vi "CPP-Multiplot.vi"(0 "PlotArray":cluster{dbl[], dbl[]}[](array[cluster]), 1 "Job Directory":path) -> (2 "Saved Automatically?":bool, 3 "gnuplotScript":string, 4 "Plot data file":path)   [LabVIEW 2014]
uses:
  gnuplotScriptComponents/plotstyle.ctl
  gnuplotScriptComponents/graphPeripherals.ctl
  gnuplotScriptComponents/minAndMax.ctl
  gnuplotScriptComponents/AutoManualNumber.ctl
  gnuplotScriptComponents/ticsAndGrids.ctl
  gnuplotScriptComponents/tics.ctl
  gnuplotScriptComponents/grids.ctl
  gnuplotScriptComponents/legendProperties.ctl
  gnuplotScriptComponents/legendAppearance.ctl
  gnuplotScriptComponents/alignment.ctl
  gnuplotScriptComponents/at.ctl
  gnuplotScriptComponents/margins.ctl
  gnuplotScriptComponents/source.ctl
  gnuplotScriptComponents/Master_Legend.ctl
  gnuplotScriptComponents/MasterPeripherals.ctl
  gnuplotScriptComponents/axisName.ctl
  Results_plotter_Global.vi
panel:
  out "Multi_Plot":bool
  in  "OpenLogfile?":bool
  in  "Show Script Editor?":bool
  in  "Tab Control":T1(tab)=enum."Appearance"
  in  "Each Graph contains:":T2=enum."Series"
  in  "Rows from:":T2=enum."Until done"
  in  "Columns from:":T2=enum."Selector 1"
  in  "Margins":T3={"Top"=2.0, "Bottom"=2.0, "Left"=2.0, "Right"=2.0}
  in  "Height (in)":dbl=7.0 min=0.5 step=0.5 format="%.1f"
  in  "Width (in)":dbl=10.0 min=0.5 step=0.5 format="%.1f"
  in  "nRows":u8=3 min=1
  in  "nCols":u8=3 min=1
  in  "ScaleAdjust":dbl=0.9 min=0.1 max=2.0 step=0.1
  in  "PlotTitlesNeed $$?":bool=TRUE
  in  "Show Channels with range of Values?":bool
  in  "ManualPlotTitles":string[](array[string])
  out "AutoPlotTitles":string[](array[string])
  in  "Individual Plot Titles":bool=TRUE
  in  "Page Title Pre Block":string
  in  "Page Title Post Block":string
  in  "Values to include in Page Title":i32[](listbox)
  in  "Plot Title Offset (characters)":cluster{"horizontal":dbl, "vertical":dbl}
  out "Final Title":string
  in  "PlotNamesNeed $$?":bool=TRUE
  in  "Plot Legends Manual":string[](array[string])
  in  "Plotstyles":T4[](array[typedef])=[{"Style"="linespoints", "Color"=16711680, "PointType"=1, "PointSize"=1.0000001, "LineWidth"=1.0, "LineType"=1}, {"Style"="linespoints", "Color"=16860, "PointType"=2, "PointSize"=1.0000001, "LineWidth"=1.0, "LineType"=1}, {"Style"="linespoints", "Color"=51228, "PointType"=3, "PointSize"=1.0, "LineWidth"=1.0, "LineType"=1}, {"Style"="linespoints", "Color"=0, "PointType"=4, "PointSize"=1.0, "LineWidth"=1.0, "LineType"=1}, {"Style"="linespoints", "Color"=9567230, "PointType"=1, "PointSize"=1.0000001, "LineWidth"=1.0, "LineType"=1}, {"Style"="linespoints", "Color"=12369084, "PointType"=1, "PointSize"=1.0000001, "LineWidth"=1.0, "LineType"=1}, {"Style"="linespoints", "Color"=15667967, "PointType"=1, "PointSize"=1.0000001, "LineWidth"=1.0, "LineType"=1}, {"Style"="linespoints", "Color"=15400704, "PointType"=1, "PointSize"=1.0000001, "LineWidth"=1.0, "LineType"=1}] caption="Style                      Colour    PointType       PointSize         Linewidth        Linestyle" {"LineType" min=1 max=6 step=1; "LineWidth" min=1 max=6 step=1; "PointSize" min=0 step=0.1}
  out "Plot Legends Auto":string[](array[string])
  out "No of Series supplied":i32
  out "No of Graph Slots Available":i32
  in  "Plot Legends":bool=TRUE
  in  "X axis label":enum32{"Autolabel", "Manual Label"}(tab)
  out "X or theta label":string
  in  "X or theta label Manual":string
  in  "LegendProperties":T5={"Appearance"={"layout"="", "text-sample order"="", "key order"="", "surroundingBox"="", "MaxRows"=0, "MaxCols"=0, "WidthAdjust"=0.0}, "Alignment"={"Horizontal"="", "Vertical"=""}, "Location"="auto", "\"At\" location"={"XcoordSys"="", "YcoordSys"="", "Xvalue"=0.0, "Yvalue"=0.0}}
  in  "Y/R tics And Grids":T9={"tics"={"ticMin"=0.0, "ticStep"=5.0, "ticMax"=0.0, "minorDivsPerMajor"=2, "ticSpacing"=enum."Auto Tics", "ticPosition"=enum."Inside, no mirror"}, "Grids"={"Gridlines"=enum."No grids", "Zeroaxis"=enum."No zero axis"}, "Mapping"=enum."Lin"}
  in  "X/Theta tics And Grids":T9={"tics"={"ticMin"=0.0, "ticStep"=5.0, "ticMax"=0.0, "minorDivsPerMajor"=2, "ticSpacing"=enum."Auto Tics", "ticPosition"=enum."Inside, no mirror"}, "Grids"={"Gridlines"=enum."Major grid", "Zeroaxis"=enum."No zero axis"}, "Mapping"=enum."Lin"}
  in  "PlotType":enum32{"XY", "Polar"}(tab)
  in  "yAxisBounds":T12={"Min"={"Auto"=TRUE, "Value"=0.0}, "Max"={"Auto"=TRUE, "Value"=0.0}}
  in  "Additional XYgnuplot":string
  in  "xAxisBounds":T12={"Min"={"Auto"=TRUE, "Value"=0.0}, "Max"={"Auto"=TRUE, "Value"=0.0}}
  in  "Set bounds using XY Plot \non Results file plotter":bool
  in  "Angle Units":bool=TRUE
  in  "AngleMode":string(combo)="Compass"
  in  "wrapGapsUpTo:":dbl=30.0 step=0.1
  in  "Additional Polar gnuplot":string
  in  "rAxisBounds":T12={"Min"={"Auto"=FALSE, "Value"=0.0}, "Max"={"Auto"=FALSE, "Value"=1.5}}
  in  "Y axis label":enum32{"Autolabel", "Manual Label"}(tab)
  out "Y or R label":string
  in  "Y or R label Manual 2":string
  in  "PeripheralsMasterControl":T14
  in  "Legend Options":T15=enum."Single Legend Below table"
  in  "GraphPeripherals":T16[][](array[typedef])
  out "PlotCommand":string
  in  "Filename Max length":i32=255
  out "File Path Control":path
  out "AuditTrail":string[](array[string])
  out "Desired Legends":string[][](array[string])
  out "original name had conflict":bool
  out "crossplatform problem":bool
  # "Rows/ Columns/ Series from: controls not wired- just a thought for explicit control of what goes where...?"
  # "Overall Page Title"
  # "There are as many graphs as there are titles (from Selector 2)...."
  # "Plot Styles"
  # "Each graph contains plots from Selector 1..."
  # "X/theta"
  # "Y/r"
  # "Shows the numbered line colours and point styles available- well it would, if it didn't disappear every time I update from the repository..!"
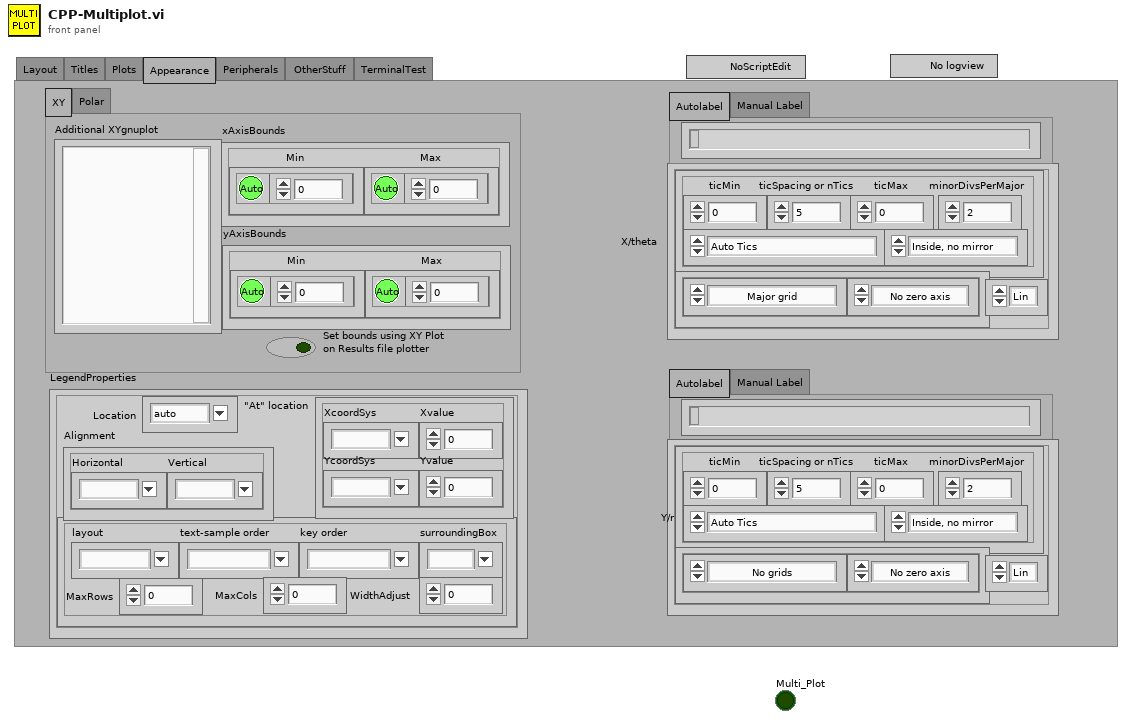
[diagram p1: front panel]
types:
  T1 = enum32{"Layout", "Titles", "Plots", "Appearance", "Peripherals", "OtherStuff ", "TerminalTest"}
  T2 = typedef "source.ctl" = enum16{"Specified:", "Selector 1", "Selector 2", "Until done", "Series"}
  T3 = typedef "margins.ctl" = cluster{"Top":dbl, "Bottom":dbl, "Left":dbl, "Right":dbl}
  T4 = typedef "plotstyle.ctl" = cluster{"Style":string, "Color":u32, "PointType":i32, "PointSize":sgl, "LineWidth":sgl, "LineType":u8}
  T5 = typedef "legendProperties.ctl" = cluster{"Appearance":T6, "Alignment":T7, "Location":string, "\"At\" location":T8}
  T6 = typedef "legendAppearance.ctl" = cluster{"layout":string, "text-sample order":string, "key order":string, "surroundingBox":string, "MaxRows":u32, "MaxCols":u32, "WidthAdjust":dbl}
  T7 = typedef "alignment.ctl" = cluster{"Horizontal":string, "Vertical":string}
  T8 = typedef "at.ctl" = cluster{"XcoordSys":string, "YcoordSys":string, "Xvalue":dbl, "Yvalue":dbl}
  T9 = typedef "ticsAndGrids.ctl" = cluster{"tics":T10, "Grids":T11, "Mapping":enum8{"Lin", "Log"}}
  T10 = typedef "tics.ctl" = cluster{"ticMin":dbl, "ticStep":dbl, "ticMax":dbl, "minorDivsPerMajor":i32, "ticSpacing":enum16{"Auto Tics", "Fixed spacing", "Fixed Minimum and Spacing", "Start, Spacing and Maximum", "Approx n Tics (rounded)"}, "ticPosition":enum16{"Inside, no mirror", "Inside, mirrored", "Outside, no mirror", "Outside, mirrored", "Invisible"}}
  T11 = typedef "grids.ctl" = cluster{"Gridlines":enum16{"No grids", "Major grid", "Minor grid", "Major and Minor"}, "Zeroaxis":enum16{"No zero axis", "Show zero axis"}}
  T12 = typedef "minAndMax.ctl" = cluster{"Min":T13, "Max":T13}
  T13 = typedef "AutoManualNumber.ctl" = cluster{"Auto":bool, "Value":dbl}
  T14 = typedef "MasterPeripherals.ctl" = enum16{"Use Table", "Titles On", "Edges Only", "All Off"}
  T15 = typedef "Master_Legend.ctl" = enum16{"No Legend", "Single Legend Below table", "Legend as per array"}
  T16 = typedef "graphPeripherals.ctl" = cluster{"title":bool, "key":bool, "Xtic":bool, "Ytic":bool, "Xlab":bool, "Ylab":bool}
  T17 = typedef "axisName.ctl" = string
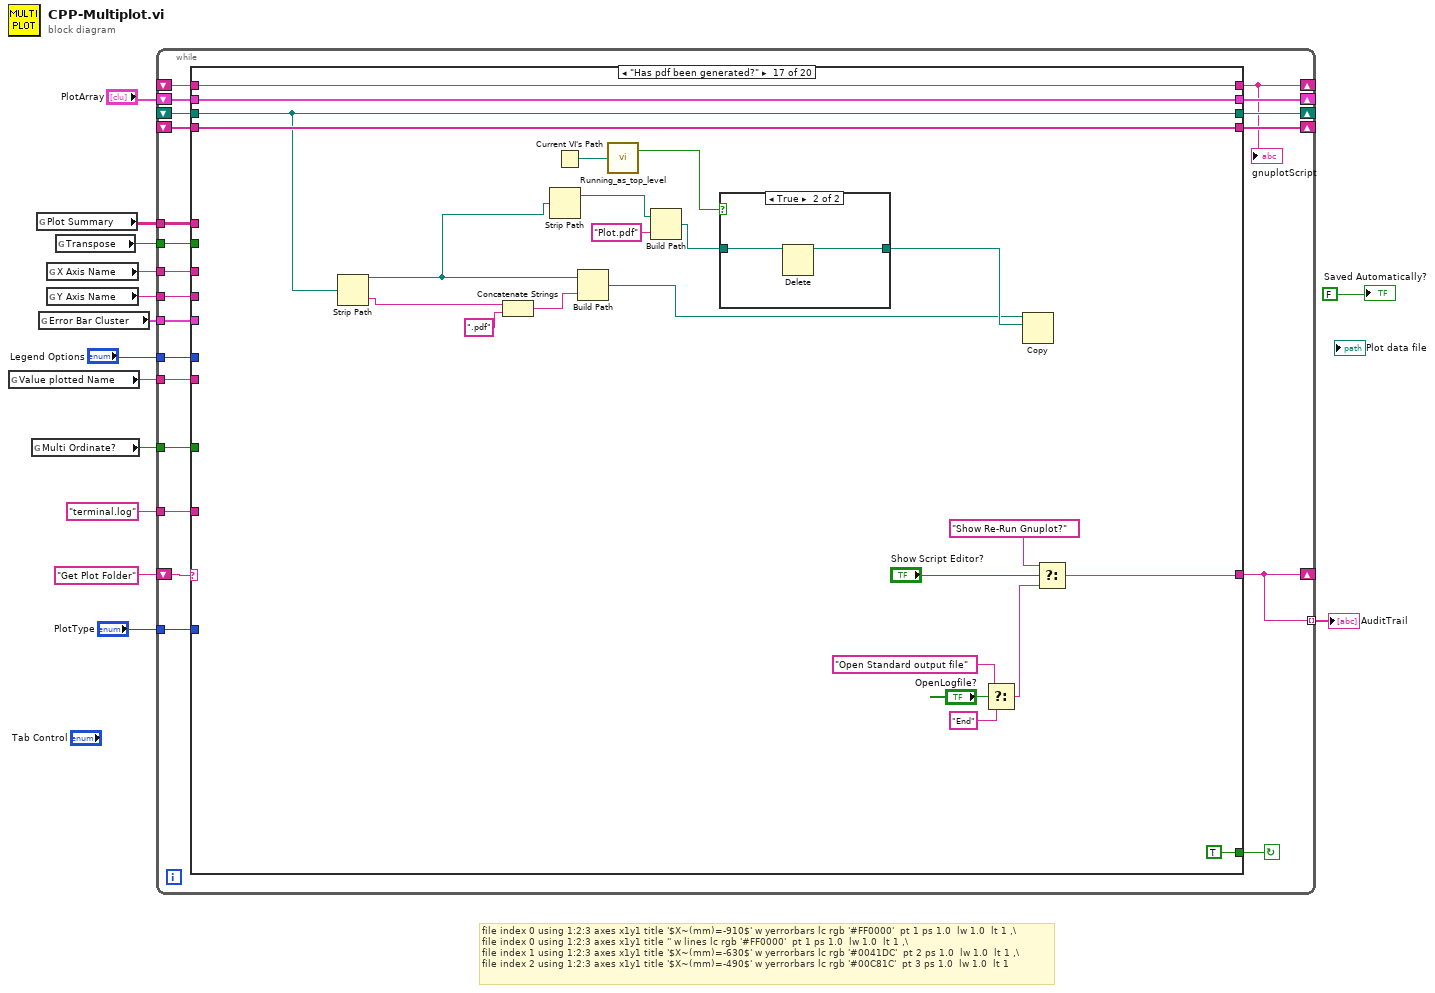
[diagram p0: block diagram]
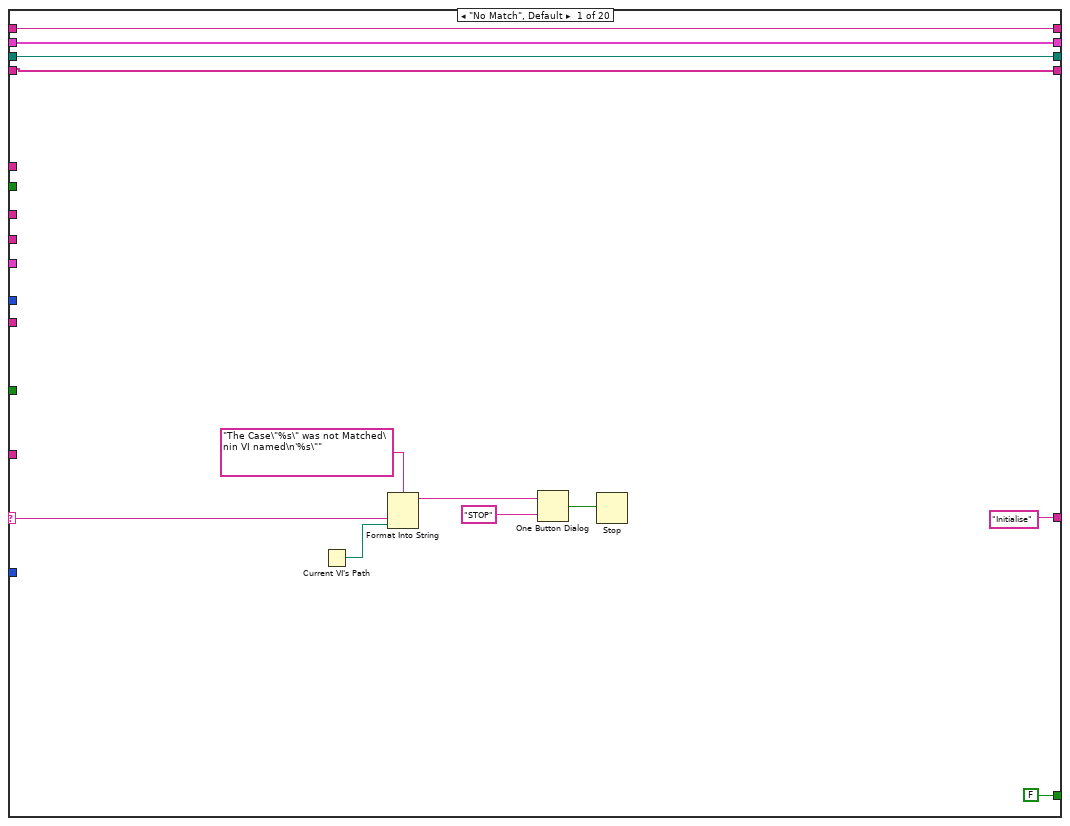
[diagram p2: hidden frame]
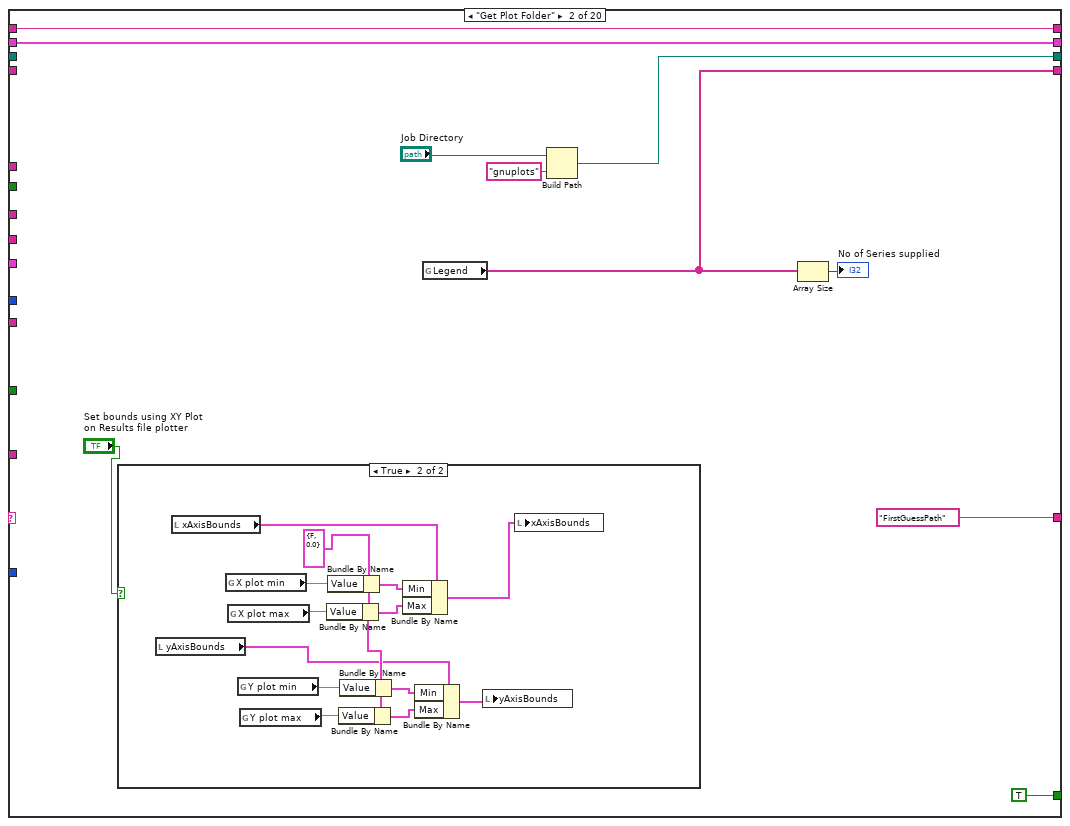
[diagram p3: hidden frame]
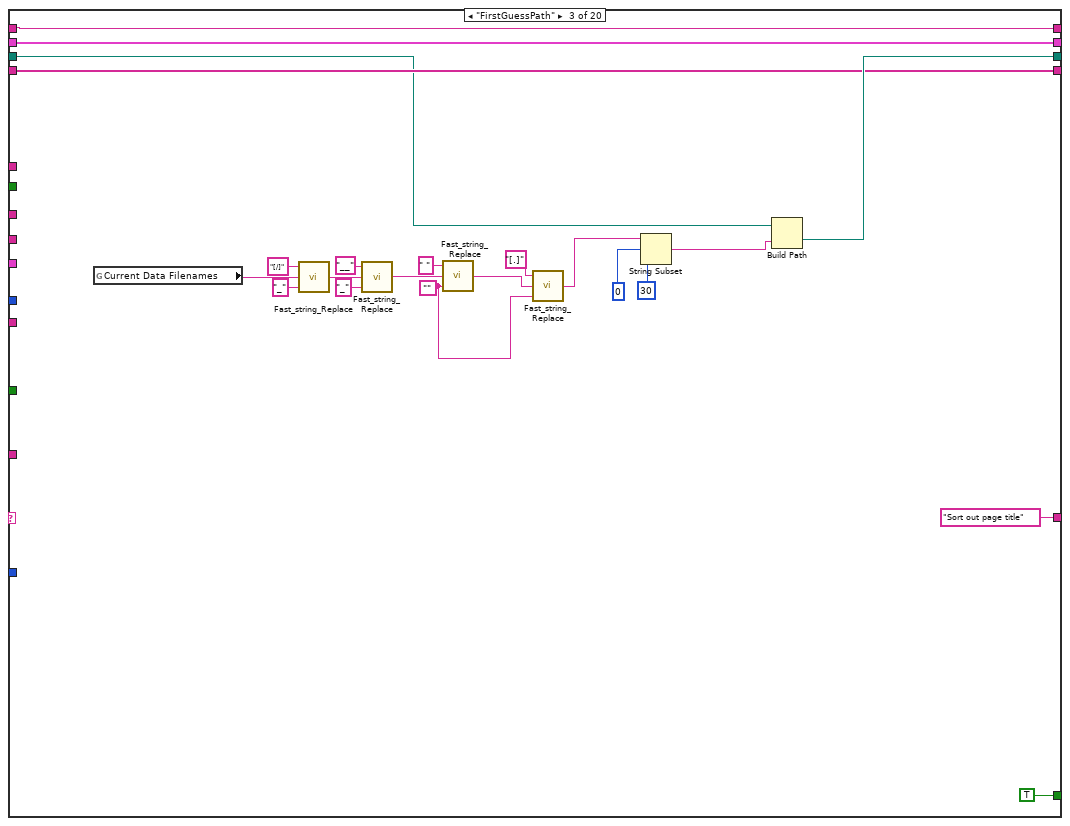
[diagram p5: hidden frame]
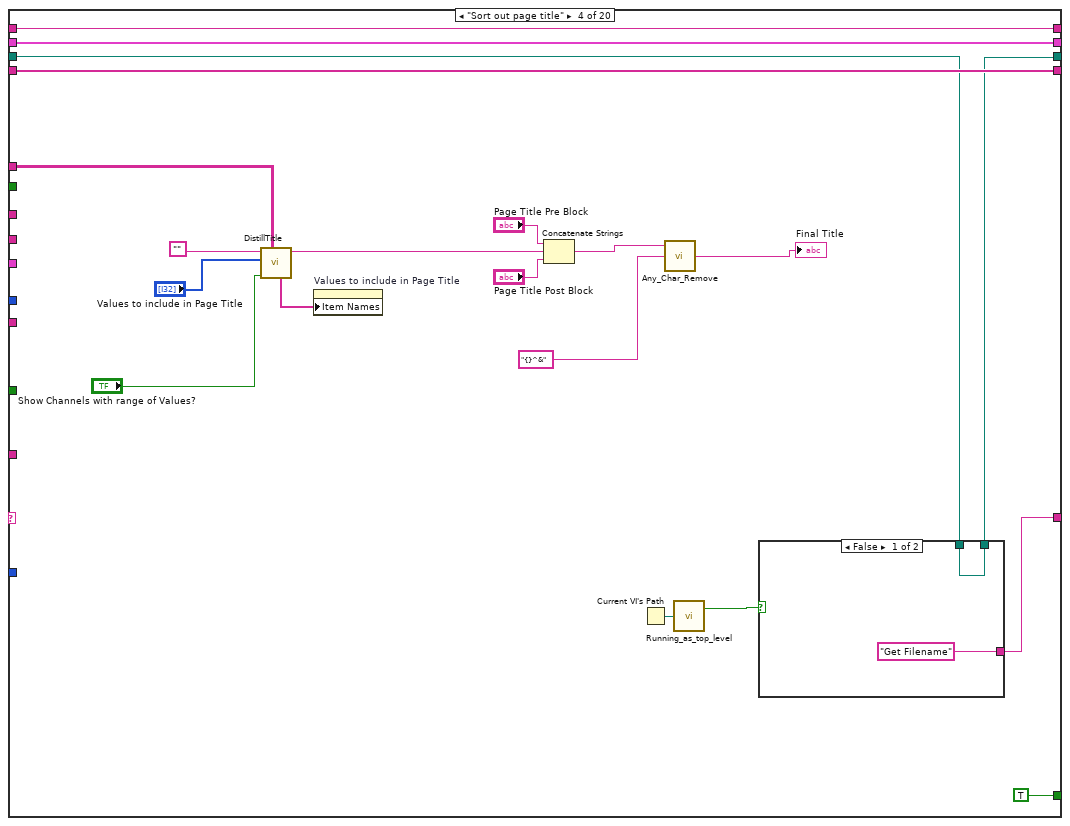
[diagram p6: hidden frame]
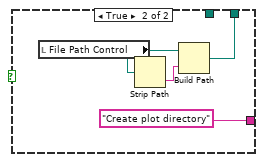
[diagram p7: hidden frame]
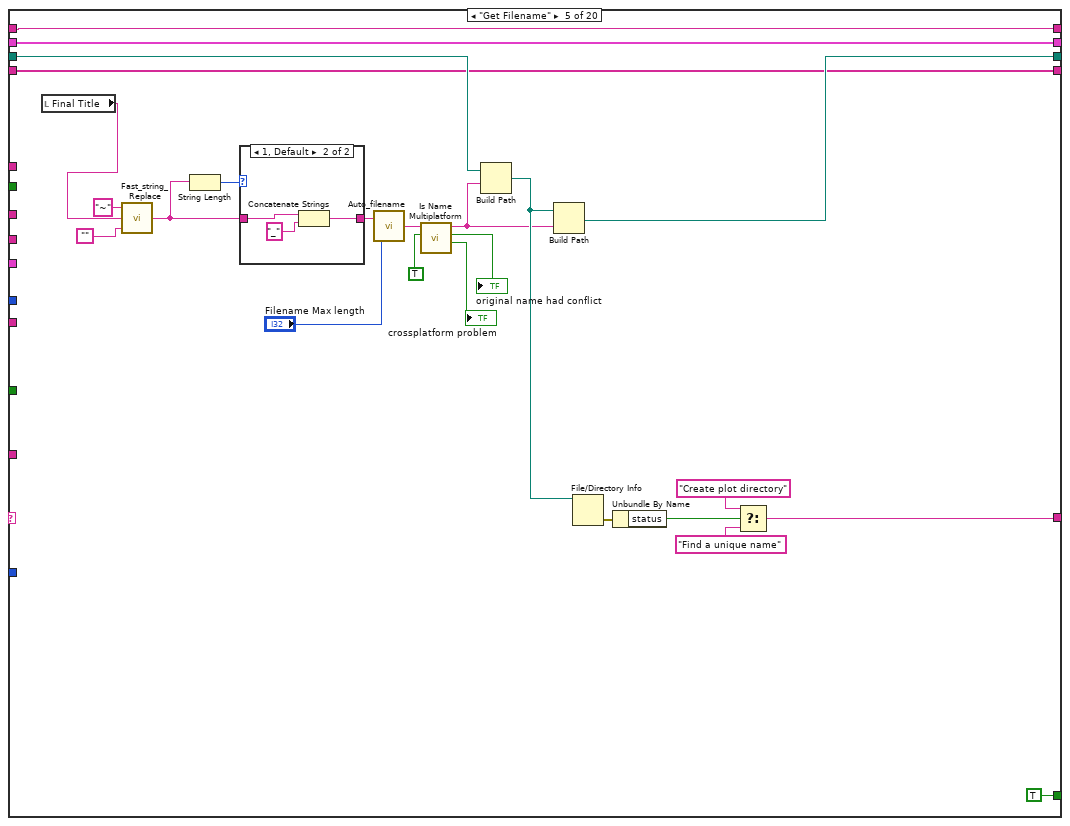
[diagram p8: hidden frame]
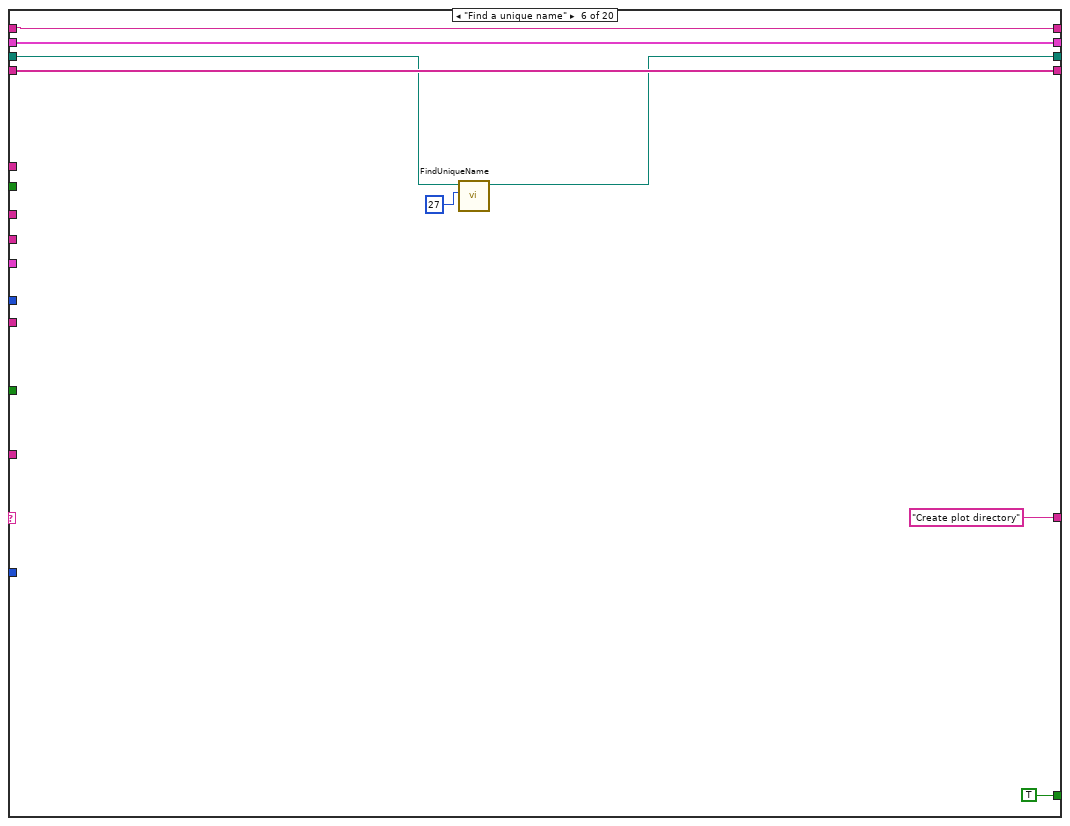
[diagram p10: hidden frame]
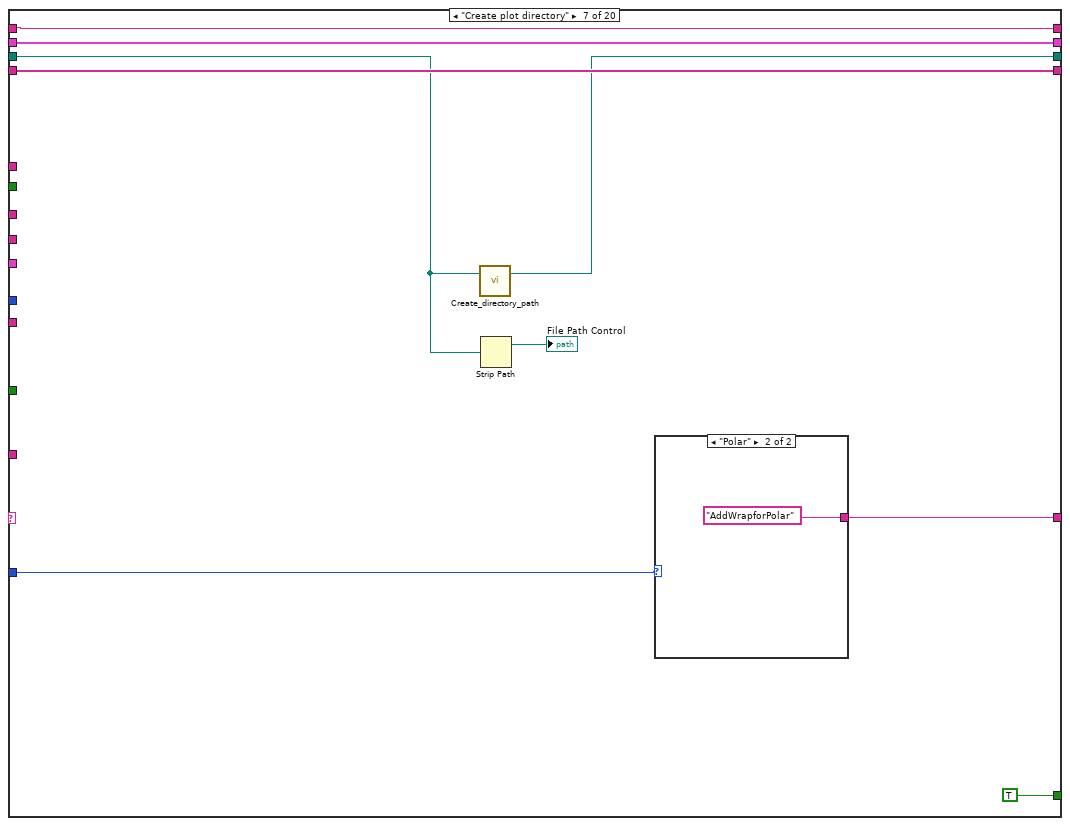
[diagram p11: hidden frame]
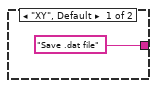
[diagram p12: hidden frame]
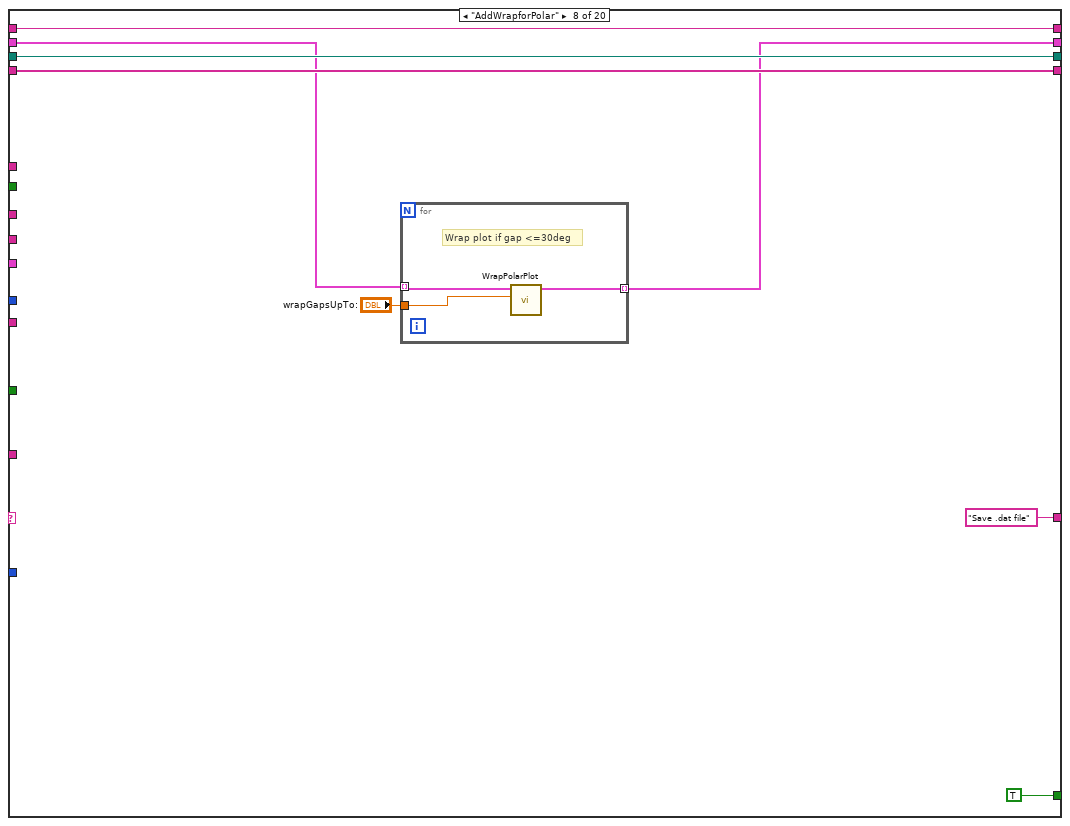
[diagram p13: hidden frame]
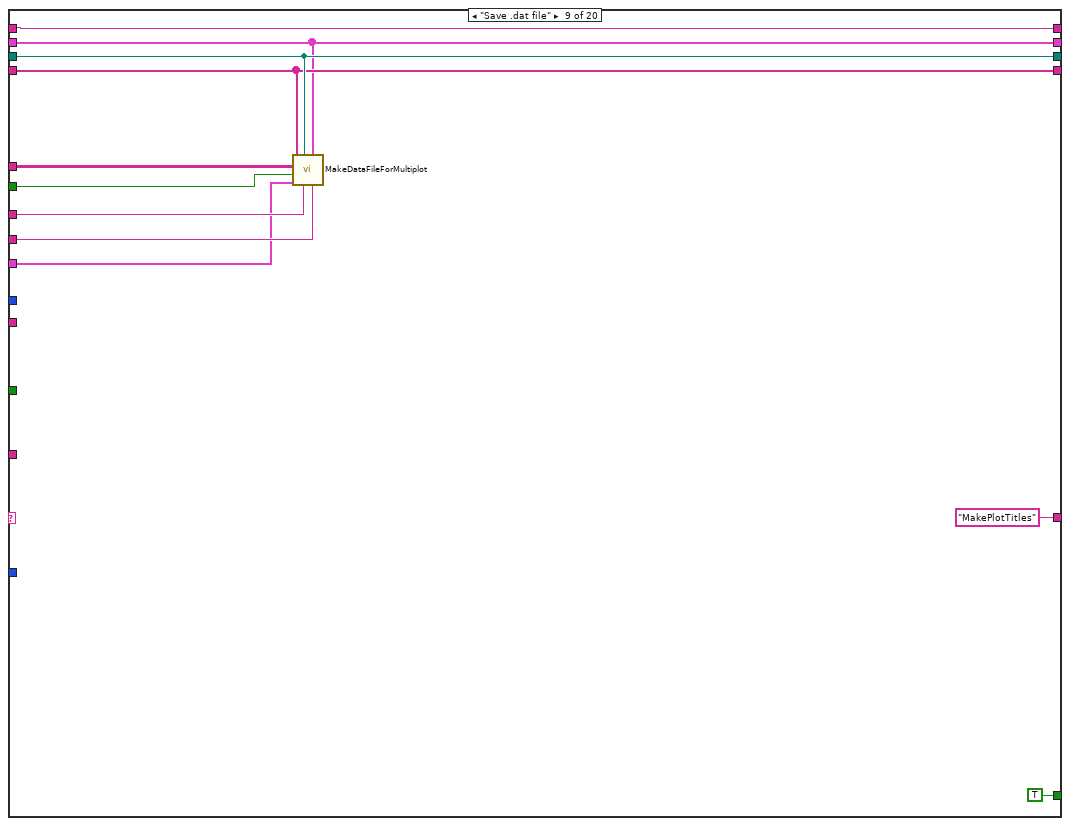
[diagram p14: hidden frame]
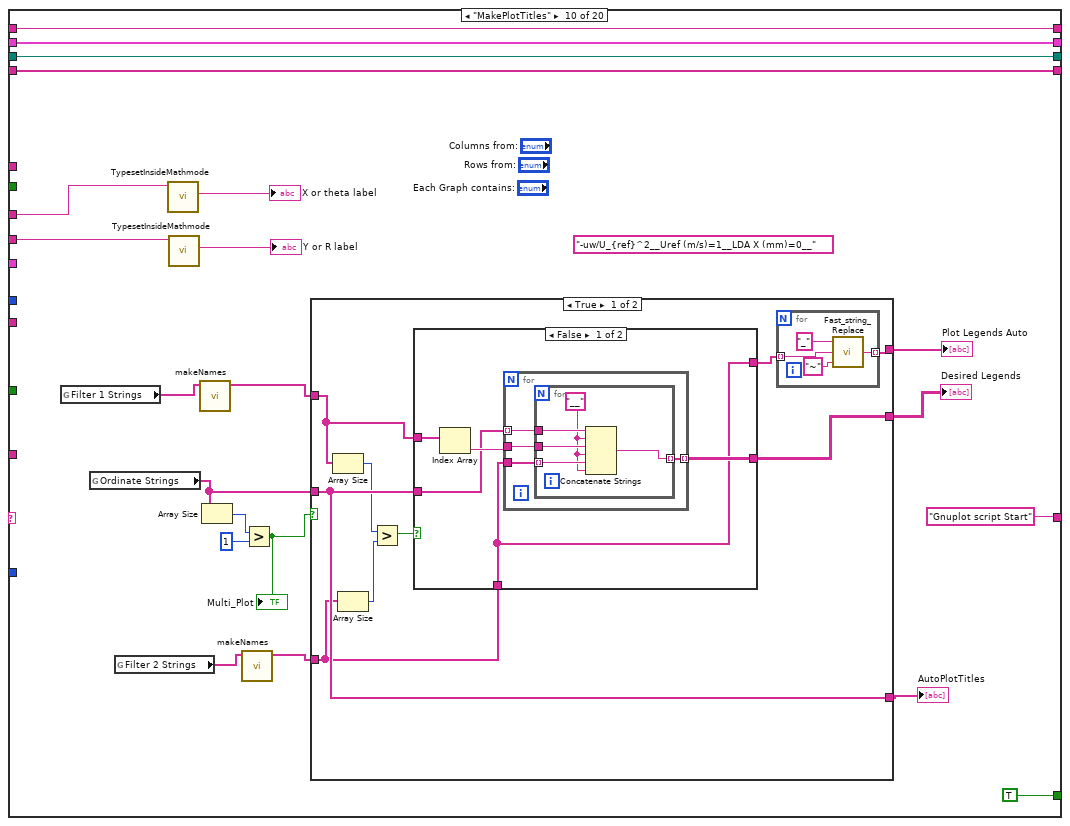
[diagram p15: hidden frame]
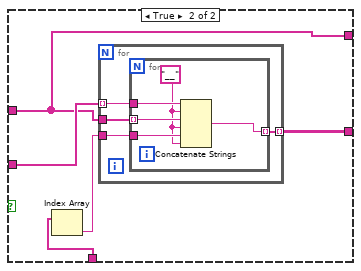
[diagram p16: hidden frame]
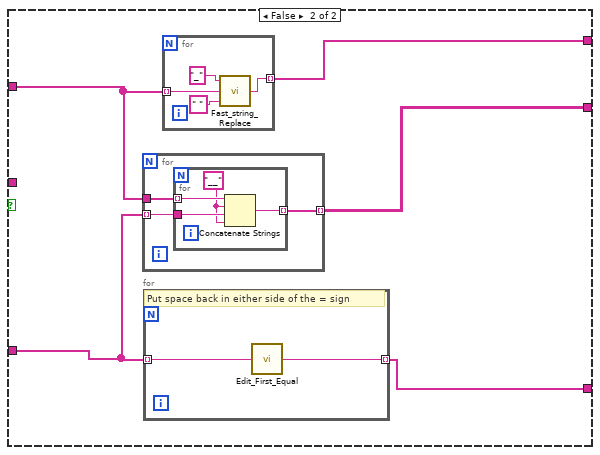
[diagram p17: hidden frame]
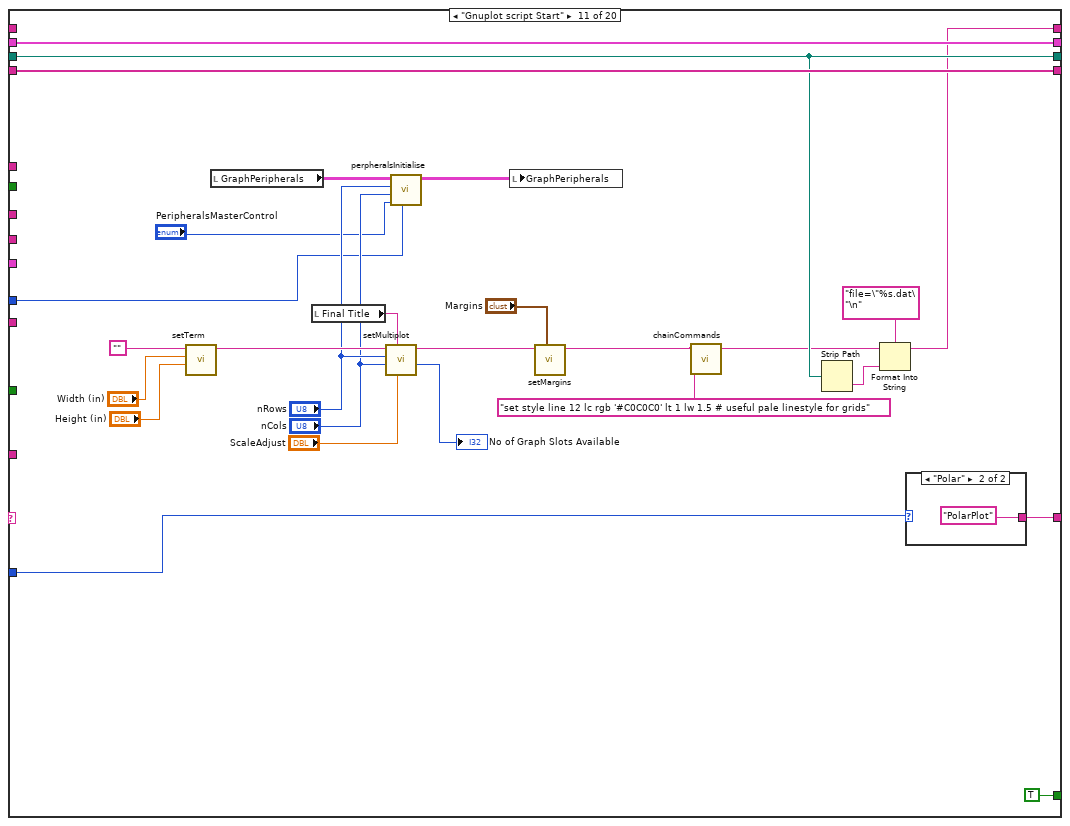
[diagram p18: hidden frame]
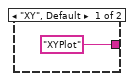
[diagram p19: hidden frame]
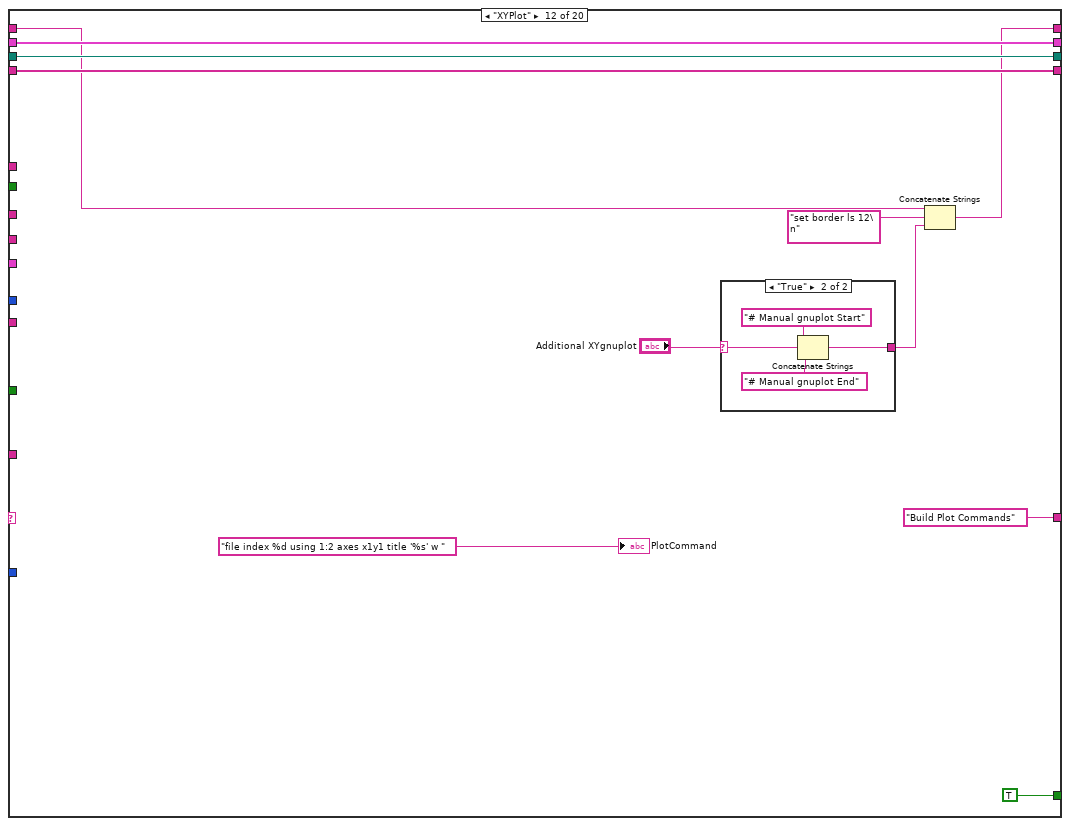
[diagram p20: hidden frame]
diagram:
  # "file index 0 using 1:2:3 axes x1y1 title '$X~(mm)=-910$' w yerrorbars lc rgb '#FF0000'  pt 1 ps 1.0  lw 1.0  lt 1 ,\\\nfile index 0 using 1:2:3 axes x1y1 title '' w lines lc rgb '#FF0000'  pt 1 ps 1.0  lw 1.0  lt 1 ,\\\nfile index 1 using 1:2:3 axes x1y1 title '$X~(mm)=-630$' w yerrorbars lc rgb '#0041DC'  pt 2 ps 1.0  lw 1.0  lt 1 ,\\\nfile index 2 using 1:2:3 axes x1y1 title '$X~(mm)=-490$' w yerrorbars lc rgb '#00C81C'  pt 3 ps 1.0  lw 1.0  lt 1"
  n1 = global read "Results_plotter_Global.vi" "Value plotted Name"() -> (w10:string)
  n2 = global read "Results_plotter_Global.vi" "Multi Ordinate?"() -> (w6:bool)
  n3 = global read "Results_plotter_Global.vi" "Plot Summary"() -> (w13:string[][])
  n4 = global read "Results_plotter_Global.vi" "Error Bar Cluster"() -> (w1:cluster{string[]}[])
  n5 = global read "Results_plotter_Global.vi" "X Axis Name"() -> (w12:string)
  n6 = global read "Results_plotter_Global.vi" "Y Axis Name"() -> (w11:string)
  n7 = global read "Results_plotter_Global.vi" "Transpose"() -> (w7:bool)
  n8 = while {
    shift-left: "Get Plot Folder" -> [w34]
    shift-right: [w18] -> _
    tunnel: w13 -> [w33]
    shift-right: [w32] -> _
    shift-left: _ -> [w31]
    tunnel: w12 -> [w30]
    tunnel: w11 -> [w29]
    tunnel: w10 -> [w28]
    shift-right: [w26] -> _
    shift-left: "PlotArray" -> [w27]
    shift-right: [w19] -> _
    shift-left: _ -> [w25]
    shift-right: [w24] -> _
    shift-left: _ -> [w23]
    tunnel: "terminal.log" -> [w22]
    tunnel: w7 -> [w21]
    tunnel: w6 -> [w20]
    tunnel: [w18] -> w5 mode=indexing
    tunnel: "PlotType" -> [w17]
    tunnel: "Legend Options" -> [w16]
    tunnel: w1 -> [w15]
    stop <- w35 continue-if-true
    n9 = case shown="\"Has pdf been generated?\"" w34 {
      selector: w34 -> [w36 _ _ _ _ _ _ _ _ _ _ _ _ _ _ _ _ _ _ _]
      tunnel: [FALSE TRUE TRUE ("Top Level") TRUE ("Top Level") TRUE ("Top Level") TRUE ("Top Level") TRUE TRUE ("Top Level") TRUE ("Top Level") TRUE ("Top Level") TRUE ("Top Level") TRUE ("Top Level") TRUE ("Top Level") TRUE ("Top Level") TRUE ("Top Level") TRUE ("Top Level") TRUE ("Top Level") FALSE ("Top Level") TRUE ("Top Level") FALSE ("Top Level")] -> w35
      tunnel: ["Initialise" "FirstGuessPath" "Sort out page title" w104 w140 "Create plot directory" w155 "Save .dat file" "MakePlotTitles" "Gnuplot script Start" w291 "Build Plot Commands" "Build Plot Commands" "Write gnuplot file" ("t") "Execute shell script" ("t") "Has pdf been generated?" ("t") w540 "End" "End" ("t") "End" ("t")] -> w18
      tunnel: w33 -> [_ _ _ w99 _ _ _ _ w185 _ _ _ _ _ _ _ _ _ _ _]
      tunnel: [w40 w55 w92 w106 w141 w147 w160 w172 w186 w208 w282 w307 w330 w382 w510 w518 w535 w552 w562 w573] -> w32
      tunnel: w31 -> [w40 _ w88 w105 w137 w148 w159 w172 w186 w208 w282 w307 w330 w382 w510 w518 w535 w552 w562 w573]
      tunnel: w30 -> [_ _ _ _ _ _ _ _ w184 w202 _ _ _ _ _ _ _ _ _ _]
      tunnel: w29 -> [_ _ _ _ _ _ _ _ w183 w201 _ _ _ _ _ _ _ _ _ _]
      tunnel: w28 -> [_ _ _ _ _ _ _ _ _ _ _ _ _ _ _ _ _ _ _ _]
      tunnel: w27 -> [w39 w51 w91 w112 w139 w151 w163 w168 w180 w207 w294 w306 w331 w348 w516 w523 w546 w557 w567 w572]
      tunnel: [w39 w51 w91 w112 w139 w151 w163 w167 w180 w207 w294 w306 w331 w348 w516 w523 w546 w557 w567 w572] -> w26
      tunnel: w25 -> [w38 w54 w90 w110 w138 w150 w162 w173 w187 w206 _ w300 w325 w374 w506 w521 w544 w555 w565 w571]
      tunnel: [w38 w54 w90 w110 w138 w150 w162 w173 w187 w206 w279 w302 w326 w380 w506 w521 w544 w555 w565 w571] -> w19
      tunnel: [w37 w50 w89 w111 w136 w149 w161 w171 w182 w205 w293 w305 w329 w381 w511 w522 w545 w556 w566 w570] -> w24
      tunnel: w23 -> [w37 _ w89 w111 w136 w149 w161 w171 w182 w205 w293 w305 w329 w381 w511 w522 w545 w556 w566 w570]
      tunnel: w22 -> [_ _ _ _ _ _ _ _ _ _ _ _ _ _ _ w517 _ _ w560 _]
      tunnel: w21 -> [_ _ _ _ _ _ _ _ w181 _ _ _ _ w344 _ _ _ _ _ _]
      tunnel: w20 -> [_ _ _ _ _ _ _ _ _ _ _ _ _ _ _ _ _ _ _ _]
      tunnel: w17 -> [_ _ _ _ _ _ w156 _ _ _ w278 _ _ w361 _ _ _ _ _ _]
      tunnel: w16 -> [_ _ _ _ _ _ _ _ _ _ w269 _ _ w347 _ _ _ _ _ _]
      tunnel: w15 -> [_ _ _ _ _ _ _ _ w177 _ _ _ _ w345 _ _ _ _ _ _]
      frame "No Match", Default {
        n10 = Current VI's Path() -> (path=w42:path)
        n11 = Format Into String(format string="The Case\"%s\" was not Matched\nin VI named\n'%s\"" ("Format String"), w36, w42) -> (resulting string=w45:string)  [unwired: 2 in, 1 out]
        n12 = One Button Dialog(message=w45, button name ("OK")="STOP") -> (true=w43:bool)
        n13 = Stop(stop? (T)=w43) -> ()
      }
      frame "Get Plot Folder" {
        n14 = case shown="True" "Set bounds using XY Plot \non Results file plotter" {
          frame False {
          }
          frame True {
            w60 = T13 {"Auto"=FALSE, "Value"=0.0} ("Min")
            n15 = local read "yAxisBounds"() -> (w59:T12)
            n16 = local read "xAxisBounds"() -> (w70:T12)
            n17 = global read "Results_plotter_Global.vi" "X plot min"() -> (w65:dbl)
            n18 = global read "Results_plotter_Global.vi" "X plot max"() -> (w66:dbl)
            n19 = global read "Results_plotter_Global.vi" "Y plot min"() -> (w64:dbl)
            n20 = global read "Results_plotter_Global.vi" "Y plot max"() -> (w63:dbl)
            n21 = Bundle By Name(cluster=w60, "Value"=w66) -> (w68:T13)
            n22 = Bundle By Name(cluster=w60, "Value"=w65) -> (w69:T13)
            n23 = Bundle By Name(cluster=w60, "Value"=w63) -> (w62:T13)
            n24 = Bundle By Name(cluster=w60, "Value"=w64) -> (w61:T13)
            n25 = Bundle By Name(cluster=w70, "Min"=w69, "Max"=w68) -> (w67:T12)
            n26 = Bundle By Name(cluster=w59, "Min"=w61, "Max"=w62) -> (w58:T12)
            n27 = local write "yAxisBounds"(w58) -> ()
            n28 = local write "xAxisBounds"(w67) -> ()
          }
        }
        n29 = global read "Results_plotter_Global.vi" "Legend"() -> (w50:string[])
        n30 = Build Path(base path="Job Directory", name or relative path="gnuplots") -> (appended path=w55:path)
        n31 = Array Size(array=w50) -> (size(s)=→"No of Series supplied":i32)
      }
      frame "FirstGuessPath" {
        w74 = ""
        n32 = global read "Results_plotter_Global.vi" "Current Data Filenames"() -> (w78:string)
        n33 = call "Fast_string_Replace.vi"("Replace match with:"="_", "Input String"=w78, "regular expression"="[/]") -> ("Output String"=w81:string)  [unwired: 2 out]
        n34 = call "Fast_string_Replace.vi"("Replace match with:"="_", "Input String"=w81, "regular expression"="__") -> ("Output String"=w79:string)  [unwired: 2 out]
        n35 = call "Fast_string_Replace.vi"("Replace match with:"=w74, "Input String"=w79, "regular expression"=" ") -> ("Output String"=w73:string)  [unwired: 2 out]
        n36 = call "Fast_string_Replace.vi"("Replace match with:"=w74, "Input String"=w73, "regular expression"="[.]") -> ("Output String"=w72:string)  [unwired: 2 out]
        n37 = String Subset(string=w72, offset (0)=0, length (rest)=30 ("length (rest)")) -> (substring=w71:string)
        n38 = Build Path(base path=w88, name or relative path=w71) -> (appended path=w92:path)
      }
      frame "Sort out page title" {
        n39 = call "DistillTitle.vi"("Plot Summary in"=w99, "Show Channels with range of Values?"="Show Channels with range of Values?", "Indices to include in Page Title"="Values to include in Page Title", "String in"="") -> ("String out"=w103:string, "AvailableVariables"=w97:string[])  [unwired: 6 in]
        n40 = property on="Values to include in Page Title" class="LstBox (strict)"("Item Names"=w97) -> ()  [unwired: 2 in, 2 out]
        n41 = Concatenate Strings("Page Title Pre Block", w103, "Page Title Post Block") -> (w96:string)
        n42 = Current VI's Path() -> (path=w109:path)
        n43 = call "Any_Char_Remove.vi"("Individual Characters to Remove"="{}^&", "String in"=w96) -> ("String out"=→"Final Title":string)  [unwired: 1 in]
        n44 = call "Running_as_top_level.vi"("Vi path name"=w109) -> ("Top Level"=w107:bool)  [unwired: 1 out]
        n45 = case shown="False" w107 {
          tunnel: [w114 w117] -> w106
          tunnel: w105 -> [w114 _]
          tunnel: ["Get Filename" ("t") "Create plot directory"] -> w104
          frame False {
          }
          frame True {
            n46 = local read "File Path Control"() -> (w116:path)
            n47 = Strip Path(path=w116) -> (name=w115:string)  [unwired: 1 out]
            n48 = Build Path(base path=w116, name or relative path=w115) -> (appended path=w117:path)
          }
        }
      }
      frame "Get Filename" {
        n49 = local read "Final Title"() -> (w126:string)
        n50 = call "Fast_string_Replace.vi"("Replace match with:"="", "Input String"=w126, "regular expression"="~") -> ("Output String"=w123:string)  [unwired: 1 in, 1 out]
        n51 = String Length(string=w123) -> (length=w128:i32)
        n52 = case shown="1, Default" w128 {
          tunnel: [w143 w144] -> w127
          tunnel: w123 -> [w143 w146]
          frame 0 {
          }
          frame 1, Default {
            n53 = Concatenate Strings(w146, "_") -> (w144:string)
          }
        }
        n54 = call "Auto_filename.vi"("Filename Max length"="Filename Max length", "Prefix"=w127) -> ("Filename"=w130:string)
        n55 = call <vilib>:"Is Name Multiplatform.vi"("name must work for all platforms (F)"=TRUE, "filename"=w130) -> ("crossplatform problem"=→"crossplatform problem":bool, "original name had conflict"=→"original name had conflict":bool, "suggested filename"=w122:string)  [unwired: 5 in, 2 out]
        n56 = Build Path(base path=w137, name or relative path=w122) -> (appended path=w134:path)
        n57 = Build Path(base path=w134, name or relative path=w122) -> (appended path=w141:path)
        n58 = File/Directory Info(path=w134) -> (error out=w135:errorcluster)  [unwired: 1 in, 6 out]
        n59 = Unbundle By Name(w135) -> ("status"=w133:bool)
        n60 = Select(t="Create plot directory", s=w133, f="Find a unique name") -> (s? t:f=w140:string)
      }
      frame "Find a unique name" {
        n61 = call "FindUniqueName.vi"("Max Length"=27, "PathIn"=w148) -> ("UniquedPath"=w147:path)  [unwired: 9 in]
      }
      frame "Create plot directory" {
        n62 = call "Create_directory_path.vi"("Path name"=w159) -> ("Path name Out"=w160:path)  [unwired: 1 in, 1 out]
        n63 = Strip Path(path=w159) -> (stripped path=→"File Path Control":path)  [unwired: 1 out]
        n64 = case shown="\"Polar\"" w156 {
          tunnel: ["Save .dat file" "AddWrapforPolar"] -> w155
          frame "XY", Default {
          }
          frame "Polar" {
          }
        }
      }
      frame "AddWrapforPolar" {
        n65 = for {
          tunnel: w168 -> [w176] mode=indexing
          tunnel: [w175] -> w167 mode=indexing
          tunnel: "wrapGapsUpTo:" -> [w174]
          # "Wrap plot if gap <=30deg"
          n66 = call "WrapPolarPlot.vi"("maxWrap"=w174, "thetaRin"=w176) -> ("thetaRout"=w175:cluster{"Angle":dbl[], "Radius":dbl[]})  [unwired: 9 in]
        }
      }
      frame "Save .dat file" {
        n67 = call "MakeDataFileForMultiplot.vi"("Y Axis Name"=w183, "Plot Array"=w180, "X Axis Name"=w184, "Path"=w186, "Error Bar Cluster"=w177, "Transpose"=w181, "Plot Summary"=w185, "Legend"=w182) -> ()  [unwired: 4 in]
      }
      frame "MakePlotTitles" {
        (unwired) "-uw/U_{ref}^2__Uref (m/s)=1__LDA X (mm)=0__"
        n68 = global read "Results_plotter_Global.vi" "Filter 1 Strings"() -> (w188:string[])
        n69 = global read "Results_plotter_Global.vi" "Ordinate Strings"() -> (w195:string[])
        n70 = global read "Results_plotter_Global.vi" "Filter 2 Strings"() -> (w191:string[])
        n71 = call "TypesetInsideMathmode.vi"("DirtyString"=w202) -> ("Mathmode String"=→"X or theta label":string)  [unwired: 8 in, 2 out]
        n72 = call "TypesetInsideMathmode.vi"("DirtyString"=w201) -> ("Mathmode String"=→"Y or R label":string)  [unwired: 8 in, 2 out]
        n73 = call "makeNames.vi"("Strings"=w188) -> ("Names"=w189:string[])  [unwired: 10 in]
        n74 = Array Size(array=w195) -> (size(s)=w194:i32)
        n75 = call "makeNames.vi"("Strings"=w191) -> ("Names"=w190:string[])  [unwired: 10 in]
        n76 = Greater?(x=w194, y=1) -> (0:w192:bool)
        "Multi_Plot" <- w192
        n77 = case shown="True" w192 {
          tunnel: w189 -> [w212 w250]
          tunnel: w190 -> [w213 w251]
          tunnel: [w209 w254] -> w198
          tunnel: [w216 w253] -> w197
          tunnel: [w217 w252] -> w196
          tunnel: w195 -> [w216 _]
          frame True {
            n78 = Array Size(array=w212) -> (size(s)=w215:i32)
            n79 = Array Size(array=w213) -> (size(s)=w214:i32)
            n80 = Greater?(x=w215, y=w214) -> (0:w211:bool)
            n81 = case shown="False" w211 {
              tunnel: [w225 w240] -> w217
              tunnel: w216 -> [w224 w239]
              tunnel: w213 -> [w222 w238]
              tunnel: w212 -> [w223 w236]
              tunnel: [w222 w236] -> w210
              frame False {
                n82 = Index Array(array=w223) -> (element=w226:string)  [unwired: 1 in]
                n83 = for {
                  tunnel: w226 -> [w230]
                  tunnel: w222 -> [w229]
                  tunnel: [w228] -> w225 mode=indexing
                  tunnel: w224 -> [w227] mode=indexing
                  n84 = for {
                    tunnel: w230 -> [w235]
                    tunnel: w229 -> [w234] mode=indexing
                    tunnel: [w233] -> w228 mode=indexing
                    tunnel: w227 -> [w232]
                    w231 = "__" ("string")
                    n85 = Concatenate Strings(w232, w231, w235, w231, w234, w231) -> (w233:string)
                  }
                }
              }
              frame True {
                n86 = Index Array(array=w238) -> (element=w237:string)  [unwired: 1 in]
                n87 = for {
                  tunnel: w236 -> [w244]
                  tunnel: w237 -> [w243]
                  tunnel: [w242] -> w240 mode=indexing
                  tunnel: w239 -> [w241] mode=indexing
                  n88 = for {
                    tunnel: w244 -> [w249] mode=indexing
                    tunnel: w243 -> [w248]
                    tunnel: [w247] -> w242 mode=indexing
                    tunnel: w241 -> [w246]
                    w245 = "__" ("string")
                    n89 = Concatenate Strings(w246, w245, w249, w245, w248, w245) -> (w247:string)
                  }
                }
              }
            }
            n90 = for {
              tunnel: w210 -> [w220] mode=indexing
              tunnel: [w219] -> w209 mode=indexing
              n91 = call "Fast_string_Replace.vi"("Replace match with:"="~", "Input String"=w220, "regular expression"="_") -> ("Output String"=w219:string)  [unwired: 1 in, 1 out]
            }
          }
          frame False {
            n92 = for {
              tunnel: w250 -> [w263]
              tunnel: w251 -> [w262] mode=indexing
              tunnel: [w261] -> w252 mode=indexing
              n93 = for {
                tunnel: w263 -> [w267] mode=indexing
                tunnel: w262 -> [w266]
                tunnel: [w264] -> w261 mode=indexing
                w265 = "__" ("string")
                n94 = Concatenate Strings(w267, w265, w266, w265) -> (w264:string)
              }
            }
            n95 = for {
              tunnel: w251 -> [w260] mode=indexing
              tunnel: [w259] -> w253 mode=indexing
              # "Put space back in either side of the = sign"
              n96 = call "Edit_First_Equal.vi"("String in"=w260) -> ("String out"=w259:string)
            }
            n97 = for {
              tunnel: w250 -> [w256] mode=indexing
              tunnel: [w255] -> w254 mode=indexing
              n98 = call "Fast_string_Replace.vi"("Replace match with:"=" ", "Input String"=w256, "regular expression"="_") -> ("Output String"=w255:string)  [unwired: 2 out]
            }
          }
        }
        "AutoPlotTitles" <- w197
        "Plot Legends Auto" <- w198
        "Desired Legends" <- w196
      }
      frame "Gnuplot script Start" {
        n99 = call "setTerm.vi"("Height (in)"="Height (in)", "Width (in)"="Width (in)", "String in"="") -> ("String out"=w287:string)  [unwired: 7 in, 1 out]
        n100 = local read "GraphPeripherals"() -> (w274:T16[][])
        n101 = local read "Final Title"() -> (w285:string)
        n102 = call "setMultiplot.vi"("ScaleAdjust"="ScaleAdjust", "OverallTitle"=w285, "Cols"="nCols", "Rows"="nRows", "String in"=w287) -> ("nGraphs"=→"No of Graph Slots Available":i32, "String out"=w286:string)  [unwired: 4 in, 1 out]
        n103 = call "perpheralsInitialise.vi"("Legend"=w269, "PeripheralsMasterControl"="PeripheralsMasterControl", "Cols"="nCols", "Rows"="nRows", "GraphPeripheralsIn"=w274) -> ("GraphPeripheralsOut"=w275:T16[][])  [unwired: 6 in]
        n104 = local write "GraphPeripherals"(w275) -> ()
        n105 = call "setMargins.vi"("Margins"="Margins", "String in"=w286) -> ("String out"=w271:string)  [unwired: 8 in, 1 out]
        n106 = call "chainCommands.vi"("Command"="set style line 12 lc rgb '#C0C0C0' lt 1 lw 1.5 # useful pale linestyle for grids", "StringIn"=w271) -> ("StringOut"=w272:string)  [unwired: 9 in]
        n107 = Strip Path(path=w282) -> (name=w281:string)  [unwired: 1 out]
        n108 = Format Into String(format string="file=\"%s.dat\"\n" ("string"), initial string=w272, w281) -> (resulting string=w279:string)  [unwired: 1 in, 1 out]
        n109 = case shown="\"Polar\"" w278 {
          tunnel: ["XYPlot" "PolarPlot"] -> w291
          frame "XY", Default {
          }
          frame "Polar" {
          }
        }
      }
      frame "XYPlot" {
        n110 = case shown="\"True\"" "Additional XYgnuplot" {
          selector: "Additional XYgnuplot" -> [w308 w312]
          tunnel: [w308 w311] -> w298
          frame "", Default {
          }
          frame "True" {
            n111 = Concatenate Strings("# Manual gnuplot Start" ("string"), w312, "# Manual gnuplot End" ("string")) -> (w311:string)
          }
        }
        n112 = Concatenate Strings(w300, "set border ls 12\n" ("input 2"), w298) -> (w302:string)
        "PlotCommand" <- "file index %d using 1:2 axes x1y1 title '%s' w " ("format string")
      }
      frame "PolarPlot" {
        n113 = case shown="\"True\"" "Additional Polar gnuplot" {
          selector: "Additional Polar gnuplot" -> [w332 w336]
          tunnel: [w332 w335] -> w313
          frame "", Default {
          }
          frame "True" {
            n114 = Concatenate Strings("# Manual gnuplot Start" ("string"), w336, "# Manual gnuplot End" ("string")) -> (w335:string)
          }
        }
        n115 = Select(t="set angles degrees\n", s="Angle Units", f="set angles radians\n") -> (s? t:f=w315:string)
        n116 = case shown="\"Math\", Default" "AngleMode" {
          tunnel: ["90-$1" ("format string") "$1" ("format string")] -> w320
          frame "Compass" {
          }
          frame "Math", Default {
          }
        }
        n117 = Concatenate Strings(w325, w315, "set polar\nset size square\n", w313) -> (w326:string)
        n118 = Concatenate Strings("file index %d using (" ("format string"), w320, "):2 axes x1y1 title '%s' w " ("format string")) -> (w319:string)
        n119 = local write "PlotCommand"(w319) -> ()
      }
      frame "Build Plot Commands" {
        n120 = local read "Desired Legends"() -> (w343:string[][])
        n121 = local read "Plot Legends Auto"() -> (w350:string[])
        n122 = Array Size(array=w343) -> (size(s)=w342:i32[])
        n123 = local read "AutoPlotTitles"() -> (w372:string[])
        n124 = case shown="\"Autolabel\", Default" "Y axis label" {
          tunnel: [w383 "Y or R label Manual 2"] -> w356
          frame "Autolabel", Default {
            n125 = local read "Y or R label"() -> (w383:string)
          }
          frame "Manual Label" {
          }
        }
        n126 = case shown="\"Autolabel\", Default" "X axis label" {
          tunnel: [w391 "X or theta label Manual"] -> w362
          frame "Autolabel", Default {
            n127 = local read "X or theta label"() -> (w391:string)
          }
          frame "Manual Label" {
          }
        }
        n128 = Index Array(array=w342) -> (element=w341:i32)  [unwired: 1 in]
        n129 = Select(t=w350, s="Plot Legends", f="Plot Legends Manual") -> (s? t:f=w349:string[])
        n130 = local read "PlotCommand"() -> (w364:string)
        n131 = case shown="Default" w361 {
          tunnel: [T17 "theta" ("Axis") T17 "x" ("Axis")] -> w359
          tunnel: [T17 "r" ("Axis") T17 "y" ("Axis")] -> w358
          tunnel: ["rAxisBounds" "yAxisBounds"] -> w360
          frame "Polar" {
          }
          frame Default {
          }
        }
        n132 = global read "Results_plotter_Global.vi" "Legend"() -> (w368:string[])
        n133 = call "serialiseArray.vi"("GraphPeripherals"="GraphPeripherals") -> ("output array"=w369:T16[])  [unwired: 10 in]
        n134 = Select(t=w372, s="Individual Plot Titles", f="ManualPlotTitles") -> (s? t:f=w346:string[])
        n135 = for {
          shift-right: [w420] -> w375
          shift-left: "\n#Begin plots\n" -> [w418]
          tunnel: w349 -> [w421]
          tunnel: "Plotstyles" -> [w422]
          tunnel: w346 -> [w414] mode=indexing
          tunnel: w369 -> [w417] mode=indexing
          tunnel: w343 -> [w416] mode=indexing
          tunnel: w368 -> [w415]
          tunnel: "LegendProperties" -> [w402]
          tunnel: "Plot Title Offset (characters)" -> [w413]
          tunnel: w364 -> [w412]
          tunnel: w362 -> [w411]
          tunnel: w360 -> [w410]
          tunnel: w359 -> [w409]
          tunnel: w358 -> [w408]
          tunnel: w356 -> [w407]
          tunnel: "Y/R tics And Grids" -> [w406]
          tunnel: "X/Theta tics And Grids" -> [w405]
          tunnel: "xAxisBounds" -> [w404]
          tunnel: w348 -> [w403]
          tunnel: w347 -> [w401]
          tunnel: w345 -> [w397]
          tunnel: w344 -> [w396]
          tunnel: w341 -> [w395]
          tunnel: "PlotNamesNeed $$?" -> [w394]
          tunnel: "PlotTitlesNeed $$?" -> [w393]
          i -> [w400]
          # "Loops once for each graph on the multiplot"
          n136 = call "BuildPlotsOneGraph.vi"("PlotCommand"=w412, "Desired Legends"=w416, "Plotstyles"=w422, "PlotNamesNeed $$?"=w394, "Plot Legends"=w421, "PlotArray"=w403, "Legend"=w415, "Error Bar Cluster"=w397) -> ("String out"=w419:string, "Xspan"=w398:cluster{"Max":dbl, "Min":dbl}, "Yspan"=w399:cluster{"Max":dbl, "Min":dbl})  [unwired: 5 in]
          n137 = stacked-sequence {
            seq-local: [w429 _] -> [_ w476]
            seq-local: [w425 _] -> [_ w475]
            tunnel: [_ w495] -> w420
            tunnel: w419 -> [_ w494]
            tunnel: w418 -> [_ w493]
            tunnel: w417 -> [w427 w492]
            tunnel: w414 -> [_ w483]
            tunnel: w413 -> [_ w481]
            tunnel: w411 -> [_ w466]
            tunnel: w410 -> [_ w474]
            tunnel: w409 -> [_ w480]
            tunnel: w408 -> [_ w479]
            tunnel: w407 -> [_ w470]
            tunnel: w406 -> [_ w478]
            tunnel: w405 -> [_ w477]
            tunnel: w404 -> [_ w473]
            tunnel: w402 -> [w428 _]
            tunnel: w401 -> [w430 _]
            tunnel: w400 -> [w424 _]
            tunnel: w399 -> [_ w471]
            tunnel: w398 -> [_ w472]
            tunnel: w396 -> [_ w465]
            tunnel: w395 -> [w423 _]
            tunnel: w393 -> [_ w463]
            frame #0 {
              n138 = Unbundle By Name(w427) -> ("key"=w426:bool)
              n139 = case shown="\"Single Legend Below table\"" w430 {
                tunnel: [w432 w436] -> w429
                tunnel: w428 -> [w432 w437]
                tunnel: w426 -> [w431 _]
                tunnel: [w431 w435] -> w425
                tunnel: w424 -> [_ w433]
                tunnel: w423 -> [_ w434]
                frame "Legend as per array", Default {
                }
                frame "Single Legend Below table" {
                  n140 = stacked-sequence {
                    seq-local: [w439 _] -> [_ w456]
                    seq-local: [w438 _] -> [_ w455]
                    tunnel: w437 -> [_ w462]
                    tunnel: w433 -> [_ w459]
                    tunnel: [_ w458] -> w436
                    tunnel: [_ w457] -> w435
                    tunnel: w434 -> [w441 _]
                    frame #0 {
                      n141 = local read "No of Graph Slots Available"() -> (w442:i32)
                      n142 = Greater?(x=w442, y=w441) -> (0:w440:bool)
                      n143 = case shown="True" w440 {
                        tunnel: [0.6 ("\"At\" location.Xvalue") w449] -> w439
                        tunnel: [-0.03 ("\"At\" location.Yvalue") w446] -> w438
                        frame False {
                        }
                        frame True {
                          n144 = local read "nCols"() -> (w453:u8)
                          n145 = local read "nRows"() -> (w447:u8)
                          n146 = Decrement(x=w453) -> (x-1=w454:u8)
                          n147 = Increment(x=w447) -> (x+1=w445:u8)
                          n148 = Divide(x=w454, y=w453) -> (x/y=w450:dbl)
                          n149 = Divide(x=1.0, y=w445) -> (x/y=w446:dbl)
                          n150 = Divide(x=0.7, y=w453) -> (x/y=w451:dbl)
                          n151 = Add(x=w450, y=w451) -> (x+y=w449:dbl)
                        }
                      }
                    }
                    frame #1 {
                      w460 = "screen" ("\"At\" location.XcoordSys")
                      # "Use \"screen\" coordinates to place legend at bottom-center\nof entire \"screen\" of graphs; update legend cluster to \nreflect this."
                      # "Only legend the first graph"
                      n152 = Equal To 0?(x=w459) -> (x = 0?=w457:bool)
                      n153 = Bundle By Name(cluster=w462, "Location"="at", "\"At\" location.XcoordSys"=w460, "\"At\" location.Xvalue"=w456, "\"At\" location.YcoordSys"=w460, "\"At\" location.Yvalue"=w455) -> (w458:T5)
                      n154 = local write "LegendProperties"(w458) -> ()
                    }
                  }
                }
              }
            }
            frame #1 {
              n155 = local read "Multi_Plot"() -> (w468:bool)
              n156 = case shown="True" w465 {
                tunnel: w470 -> [w496 w505]
                tunnel: [w496 w504] -> w469
                tunnel: w468 -> [w499 w502]
                tunnel: [w497 w501] -> w467
                tunnel: w466 -> [w498 w501]
                frame True {
                  n157 = Select(t="", s=w499, f=w498) -> (s? t:f=w497:string)
                }
                frame False {
                  n158 = Select(t="", s=w502, f=w505) -> (s? t:f=w504:string)
                }
              }
              n159 = Unbundle By Name(w492) -> ("title"=w491:bool, "Xtic"=w487:bool, "Xlab"=w486:bool, "Ytic"=w485:bool, "Ylab"=w484:bool)
              n160 = call "TypesetInsideMathmode.vi"("Needs $$?"=w463, "DirtyString"=w483) -> ("ChosenStringtype"=w464:string)  [unwired: 7 in, 2 out]
              n161 = call "setTitle.vi"("Offset"=w481, "Set?"=w491, "Title"=w464, "String in"=w493) -> ("String out"=w490:string)  [unwired: 6 in, 1 out]
              n162 = call "setKey.vi"("LegendProperties"=w476, "Set?"=w475, "String in"=w490) -> ("String out"=w489:string)  [unwired: 7 in, 1 out]
              n163 = call "AxisControl.vi"("String in"=w489, "AxisBounds"=w473, "ticsAndGrids"=w477, "Axis"=w480, "ShowNumbers?"=w487, "ShowLabel?"=w486, "Axis Label"=w467, "DataSpan"=w472) -> ("String out"=w482:string)  [unwired: 6 in, 1 out]
              n164 = call "AxisControl.vi"("String in"=w482, "AxisBounds"=w474, "ticsAndGrids"=w478, "Axis"=w479, "ShowNumbers?"=w485, "ShowLabel?"=w484, "Axis Label"=w469, "DataSpan"=w471) -> ("String out"=w488:string)  [unwired: 6 in, 1 out]
              n165 = Concatenate Strings(w488, w494) -> (w495:string)
            }
          }
        }
        n166 = Concatenate Strings(w374, w375, "\nunset multiplot\n") -> (w380:string)
      }
      frame "Write gnuplot file" {
        w513 = FALSE  # append to file? (new file:F)
        w514 = FALSE  # advisory dialog? (display:T)
        n167 = Strip Path(path=w510) -> (stripped path=w507:path)  [unwired: 1 out]
        n168 = Build Path(base path=w507, name or relative path="gnuplot_script.txt") -> (appended path=w515:path)
        n169 = call "Write_Characters_To_File.vi"("file path (dialog if empty)"=w515, "advisory dialog? (display:T)"=w514, "character string"=w506, "append to file? (new file:F)"=w513) -> ()  [unwired: 1 in, 4 out]
      }
      frame "Execute shell script" {
        n170 = call "Run_Gnuplot_Script.vi"("logfileName"=w517, "workingDirectory"=w518) -> ()
      }
      frame "Has pdf been generated?" {
        n171 = Strip Path(path=w535) -> (stripped path=w531:path, name=w534:string)
        n172 = Concatenate Strings(w534, ".pdf" ("string")) -> (w532:string)
        n173 = Strip Path(path=w531) -> (stripped path=w530:path)  [unwired: 1 out]
        n174 = Current VI's Path() -> (path=w526:path)
        n175 = Build Path(base path=w531, name or relative path=w532) -> (appended path=w524:path)
        n176 = call "Running_as_top_level.vi"("Vi path name"=w526) -> ("Top Level"=w525:bool)  [unwired: 1 out]
        n177 = Build Path(base path=w530, name or relative path="Plot.pdf") -> (appended path=w528:path)
        n178 = case shown="True" w525 {
          tunnel: w528 -> [w548 w550]
          tunnel: [w547 w549] -> w527
          frame False {
            n179 = call "Find_Unique_Filename.vi"("Path In"=w548) -> ("Unique Path Out"=w547:path)  [unwired: 2 in]
          }
          frame True {
            n180 = Delete(path (use dialog)=w550) -> (deleted path=w549:path)  [unwired: 4 in, 2 out]
          }
        }
        n181 = Select(t="Open Standard output file" ("f"), s="OpenLogfile?", f="End") -> (s? t:f=w536:string)
        n182 = Copy(10:w527, 11:w524) -> ()  [unwired: 3 in, 3 out]
        n183 = Select(t="Show Re-Run Gnuplot?", s="Show Script Editor?", f=w536) -> (s? t:f=w540:string)
      }
      frame "Show Re-Run Gnuplot?" {
        n184 = Strip Path(path=w552) -> (stripped path=w551:path)  [unwired: 1 out]
        n185 = call "Re_run_Gnuplot.vi"("Plot folder (dialog if empty)"=w551) -> ()  [unwired: 4 out]
      }
      frame "Open Standard output file" {
        n186 = Strip Path(path=w562) -> (stripped path=w559:path)  [unwired: 1 out]
        n187 = Format Into String(format string="open \"%s\"", w560) -> (resulting string=w558:string)  [unwired: 2 in, 1 out]
        n188 = call <vilib>:"System Exec.vi"("working directory"=w559, "command line"=w558) -> ()  [unwired: 4 in, 6 out]
      }
      frame "End" {
      }
    }
    "gnuplotScript" <- w19
  }
  "AuditTrail" <- w5
  "Saved Automatically?" <- FALSE
